vi "S4GUI.vi"(7 "Tab ObsEng":enum32{"Obs", "CCD modes", "Guider", "Eng"}(tab)) -> ()   [LabVIEW 2018] (continued)
                    n2231 = call-dynamic "save config.vi"("error in (no error)"=w4233, "file config"="lastsaved.cfg", "Channel in"=w4227) -> ("error out"=w4232:errorcluster, "Channel out"=w4226:refnum<class "Channel.lvclass">)  [unwired: 7 in]
                    n2232 = call-dynamic "Read State Machine.vi"("error in (no error)"=w4232, "Device in"=w4226) -> ("error out"=w4236:errorcluster, "State Machine.lvclass"=w4224:refnum<class "State Machine.lvclass">, "Device out"=w4225:refnum<class "Channel.lvclass">)  [unwired: 7 in]
                    n2233 = call-dynamic "Write State.vi"("error in (no error)"=w4236, "State"=60, "State Machine in"=w4224) -> ("error out"=w4235:errorcluster, "State Machine out"=w4223:refnum<class "State Machine.lvclass">)  [unwired: 7 in]
                    n2234 = call-dynamic "Write State Machine.vi"("error in (no error)"=w4235, "State Machine.lvclass"=w4223, "Device in"=w4225) -> ("error out"=w4221:errorcluster, "Device out"=w4222:refnum<class "Channel.lvclass">)  [unwired: 7 in]
                    n2235 = call-dynamic "Write Channel.vi"("error in (no error)"=w4221, "Channel.lvclass"=w4222, "Acquisition in"=w4252) -> ("error out"=w4217:errorcluster, "Acquisition out"=w4218:refnum<class "Acquisition.lvclass">)  [unwired: 7 in]
                  }
                }
                n2236 = call-dynamic "Write AcquisitionA.vi"("error in (no error)"=w4188, "Acquisition.lvclass"=w4189, "S4ACS_GUI in"=w4190) -> ("error out"=w4179:errorcluster, "S4ACS_GUI out"=w4194:refnum<class "S4GUI.lvclass">)  [unwired: 7 in]
                n2237 = call "Write AcquisitionB.vi"("error in (no error)"=w4186, "Acquisition.lvclass"=w4187, "S4ACS_GUI in"=w4194) -> ("error out"=w4178:errorcluster, "S4ACS_GUI out"=w4193:refnum<class "S4GUI.lvclass">)  [unwired: 7 in]
                n2238 = call-dynamic "Write AcquisitionC.vi"("error in (no error)"=w4184, "Acquisition.lvclass"=w4185, "S4ACS_GUI in"=w4193) -> ("error out"=w4177:errorcluster, "S4ACS_GUI out"=w4192:refnum<class "S4GUI.lvclass">)  [unwired: 7 in]
                n2239 = call-dynamic "Write AcquisitionD.vi"("error in (no error)"=w4182, "Acquisition.lvclass"=w4183, "S4ACS_GUI in"=w4192) -> ("error out"=w4176:errorcluster, "S4ACS_GUI out"=w4191:refnum<class "S4GUI.lvclass">)  [unwired: 7 in]
                n2240 = Merge Errors(w4179, w4178, w4177, w4176) -> (w4175:errorcluster)
              }
            }
            n2241 = call-dynamic "Read prev ciclos.vi"("error in (no error)"=w4162, "S4GUI in"=w4163) -> ("error out"=w4160:errorcluster, "prev ciclos"=w4159:u32, "S4GUI out"=w4161:refnum<class "S4GUI.lvclass">)  [unwired: 7 in]
            n2242 = property on="#Cycles Done" class="Slide (strict)"("Scale.Maximum"=w4159, "Scale.Minimum"=0.0 ("Scale.Range:Minimum")) -> ()  [unwired: 2 in, 2 out]
            n2243 = local write "# Cycles"(w4159) -> ()
          }
          frame 0, Default {
            # "Async mode: Os canais são configurados com Trigger Interno para Fotometria ou Trigger Externo para Polarimetria (independentemente do status do SyncBox)"
            # "Aynchronous:"
            n2244 = call-dynamic "Read AcquisitionC.vi"("error in (no error)"=w4394, "S4ACS_GUI in"=w4393) -> ("error out"=w4398:errorcluster, "Acquisition.lvclass"=w4397:refnum<class "Acquisition.lvclass">)  [unwired: 7 in, 1 out]
            n2245 = call "Read AcquisitionB.vi"("error in (no error)"=w4394, "S4ACS_GUI in"=w4393) -> ("error out"=w4399:errorcluster, "Acquisition.lvclass"=w4400:refnum<class "Acquisition.lvclass">)  [unwired: 7 in, 1 out]
            n2246 = call-dynamic "Read AcquisitionA.vi"("error in (no error)"=w4394, "S4ACS_GUI in"=w4393) -> ("error out"=w4401:errorcluster, "Acquisition.lvclass"=w4402:refnum<class "Acquisition.lvclass">, "S4ACS_GUI out"=w4383:refnum<class "S4GUI.lvclass">)  [unwired: 7 in]
            n2247 = case shown="True" w4374 {
              tunnel: [u8 0 ("SHUTTER_MODE") w4417] -> w4373
              tunnel: w4372 -> [_ w4420]
              frame False {
                # "Fotom."
                # "Internal"
              }
              frame True {
                # "exp mode?"
                # "Internal"
                # "Polar."
                # "Ext. Start"
                n2248 = Select(t=u8 0, s=w4420, f=u8 6 ("SHUTTER_MODE")) -> (s? t:f=w4417:u8)
              }
            }
            n2249 = call-dynamic "Read AcquisitionD.vi"("error in (no error)"=w4394, "S4ACS_GUI in"=w4393) -> ("error out"=w4395:errorcluster, "Acquisition.lvclass"=w4396:refnum<class "Acquisition.lvclass">)  [unwired: 7 in, 1 out]
            n2250 = call "Read connection.vi"("error in (no error)"=w4398, "Server in"=w4397) -> ("error out"=w4407:errorcluster, "connection"=w4406:bool, "Server out"=w4408:refnum<class "Acquisition.lvclass">)  [unwired: 7 in]
            n2251 = call "Read connection.vi"("error in (no error)"=w4399, "Server in"=w4400) -> ("error out"=w4410:errorcluster, "connection"=w4409:bool, "Server out"=w4411:refnum<class "Acquisition.lvclass">)  [unwired: 7 in]
            n2252 = call "Read connection.vi"("error in (no error)"=w4395, "Server in"=w4396) -> ("error out"=w4404:errorcluster, "connection"=w4403:bool, "Server out"=w4405:refnum<class "Acquisition.lvclass">)  [unwired: 7 in]
            n2253 = call "Read connection.vi"("error in (no error)"=w4401, "Server in"=w4402) -> ("error out"=w4413:errorcluster, "connection"=w4412:bool, "Server out"=w4414:refnum<class "Acquisition.lvclass">)  [unwired: 7 in]
            n2254 = case shown="True" w4406 {
              tunnel: w4408 -> [w4465 w4476]
              tunnel: w4407 -> [w4464 w4475]
              tunnel: [w4465 w4474] -> w4378
              tunnel: [w4464 w4473] -> w4377
              tunnel: w4373 -> [_ w4472]
              frame False {
              }
              frame True {
                # "nome do arquivo .cfg"
                # "seção no arquivo .cfg"
                n2255 = call-dynamic "Read Channel.vi"("error in (no error)"=w4475, "Acquisition in"=w4476) -> ("error out"=w4480:errorcluster, "Channel.lvclass"=w4479:refnum<class "Channel.lvclass">, "Acquisition out"=w4478:refnum<class "Acquisition.lvclass">)  [unwired: 7 in]
                n2256 = call-dynamic "Read Interface.vi"("error in (no error)"=w4480, "Channel in"=w4479) -> ("error out"=w4487:errorcluster, "Interface.lvclass"=w4488:refnum<class "Interface.lvclass">, "Channel out"=w4477:refnum<class "Channel.lvclass">)  [unwired: 7 in]
                n2257 = call-dynamic "Get CCD_Config.vi"("error in (no error)"=w4487, "Interface in"=w4488) -> ("error out"=w4485:errorcluster, "output cluster"=w4484:T31, "Interface out"=w4489:refnum<class "Interface.lvclass">)  [unwired: 7 in]
                n2258 = Bundle By Name(cluster=w4484, "TRIGGER_MODE"=w4472) -> (w4486:T31)
                n2259 = call-dynamic "Set CCD_Config.vi"("error in (no error)"=w4485, "input cluster"=w4486, "Interface in"=w4489) -> ("error out"=w4483:errorcluster, "Interface out"=w4490:refnum<class "Interface.lvclass">)  [unwired: 7 in]
                n2260 = Flatten To String(anything=w4486, error in (no error)=w4483) -> (data string=w4481:string, error out=w4482:errorcluster)  [unwired: 2 in, 1 out]
                n2261 = call "Write flatted cluster.vi"("error in (no error)"=w4482, "flatted cluster"=w4481, "Interface in"=w4490) -> ("error out"=w4492:errorcluster, "Interface out"=w4491:refnum<class "Interface.lvclass">)  [unwired: 7 in]
                n2262 = call-dynamic "Write Interface.vi"("error in (no error)"=w4492, "Interface.lvclass"=w4491, "Channel in"=w4477) -> ("error out"=w4498:errorcluster, "Channel out"=w4499:refnum<class "Channel.lvclass">)  [unwired: 7 in]
                n2263 = call "Write section_name.vi"("error in (no error)"=w4498, "section_name"="CCD_ACS3", "Channel in"=w4499) -> ("error out"=w4496:errorcluster, "Channel out"=w4502:refnum<class "Channel.lvclass">)  [unwired: 7 in]
                n2264 = call-dynamic "save config.vi"("error in (no error)"=w4496, "file config"="lastsaved.cfg", "Channel in"=w4502) -> ("error out"=w4497:errorcluster, "Channel out"=w4503:refnum<class "Channel.lvclass">)  [unwired: 7 in]
                n2265 = call-dynamic "Read State Machine.vi"("error in (no error)"=w4497, "Device in"=w4503) -> ("error out"=w4493:errorcluster, "State Machine.lvclass"=w4505:refnum<class "State Machine.lvclass">, "Device out"=w4504:refnum<class "Channel.lvclass">)  [unwired: 7 in]
                n2266 = call-dynamic "Write State.vi"("error in (no error)"=w4493, "State"=60, "State Machine in"=w4505) -> ("error out"=w4494:errorcluster, "State Machine out"=w4506:refnum<class "State Machine.lvclass">)  [unwired: 7 in]
                n2267 = call-dynamic "Write State Machine.vi"("error in (no error)"=w4494, "State Machine.lvclass"=w4506, "Device in"=w4504) -> ("error out"=w4470:errorcluster, "Device out"=w4471:refnum<class "Channel.lvclass">)  [unwired: 7 in]
                n2268 = call-dynamic "Read prev ciclos.vi"("error in (no error)"=w4470, "Channel in"=w4471) -> ("error out"=w4468:errorcluster, "prev ciclos"=w4466:u32, "Channel out"=w4469:refnum<class "Channel.lvclass">)  [unwired: 7 in]
                n2269 = local write "#cycles ch3"(w4466) -> ()
                n2270 = property on="Cycles Done ch3" class="Slide (strict)"("Scale.Maximum"=w4466, "Scale.Minimum"=0.0 ("Scale.Range:Minimum")) -> ()  [unwired: 2 in, 2 out]
                n2271 = call-dynamic "Write Channel.vi"("error in (no error)"=w4468, "Channel.lvclass"=w4469, "Acquisition in"=w4478) -> ("error out"=w4473:errorcluster, "Acquisition out"=w4474:refnum<class "Acquisition.lvclass">)  [unwired: 7 in]
              }
            }
            n2272 = case shown="True" w4403 {
              tunnel: w4405 -> [w4422 w4433]
              tunnel: w4404 -> [w4421 w4432]
              tunnel: [w4422 w4431] -> w4376
              tunnel: [w4421 w4430] -> w4375
              tunnel: w4373 -> [_ w4429]
              frame False {
              }
              frame True {
                # "nome do arquivo .cfg"
                # "seção no arquivo .cfg"
                n2273 = call-dynamic "Read Channel.vi"("error in (no error)"=w4432, "Acquisition in"=w4433) -> ("error out"=w4460:errorcluster, "Channel.lvclass"=w4461:refnum<class "Channel.lvclass">, "Acquisition out"=w4462:refnum<class "Acquisition.lvclass">)  [unwired: 7 in]
                n2274 = call-dynamic "Read Interface.vi"("error in (no error)"=w4460, "Channel in"=w4461) -> ("error out"=w4453:errorcluster, "Interface.lvclass"=w4452:refnum<class "Interface.lvclass">, "Channel out"=w4463:refnum<class "Channel.lvclass">)  [unwired: 7 in]
                n2275 = call-dynamic "Get CCD_Config.vi"("error in (no error)"=w4453, "Interface in"=w4452) -> ("error out"=w4455:errorcluster, "output cluster"=w4456:T31, "Interface out"=w4451:refnum<class "Interface.lvclass">)  [unwired: 7 in]
                n2276 = Bundle By Name(cluster=w4456, "TRIGGER_MODE"=w4429) -> (w4454:T31)
                n2277 = call-dynamic "Set CCD_Config.vi"("error in (no error)"=w4455, "input cluster"=w4454, "Interface in"=w4451) -> ("error out"=w4457:errorcluster, "Interface out"=w4450:refnum<class "Interface.lvclass">)  [unwired: 7 in]
                n2278 = Flatten To String(anything=w4454, error in (no error)=w4457) -> (data string=w4459:string, error out=w4458:errorcluster)  [unwired: 2 in, 1 out]
                n2279 = call "Write flatted cluster.vi"("error in (no error)"=w4458, "flatted cluster"=w4459, "Interface in"=w4450) -> ("error out"=w4448:errorcluster, "Interface out"=w4449:refnum<class "Interface.lvclass">)  [unwired: 7 in]
                n2280 = call-dynamic "Write Interface.vi"("error in (no error)"=w4448, "Interface.lvclass"=w4449, "Channel in"=w4463) -> ("error out"=w4442:errorcluster, "Channel out"=w4441:refnum<class "Channel.lvclass">)  [unwired: 7 in]
                n2281 = call "Write section_name.vi"("error in (no error)"=w4442, "section_name"="CCD_ACS4", "Channel in"=w4441) -> ("error out"=w4444:errorcluster, "Channel out"=w4438:refnum<class "Channel.lvclass">)  [unwired: 7 in]
                n2282 = call-dynamic "save config.vi"("error in (no error)"=w4444, "file config"="lastsaved.cfg", "Channel in"=w4438) -> ("error out"=w4443:errorcluster, "Channel out"=w4437:refnum<class "Channel.lvclass">)  [unwired: 7 in]
                n2283 = call-dynamic "Read State Machine.vi"("error in (no error)"=w4443, "Device in"=w4437) -> ("error out"=w4447:errorcluster, "State Machine.lvclass"=w4435:refnum<class "State Machine.lvclass">, "Device out"=w4436:refnum<class "Channel.lvclass">)  [unwired: 7 in]
                n2284 = call-dynamic "Write State.vi"("error in (no error)"=w4447, "State"=60, "State Machine in"=w4435) -> ("error out"=w4446:errorcluster, "State Machine out"=w4434:refnum<class "State Machine.lvclass">)  [unwired: 7 in]
                n2285 = call-dynamic "Write State Machine.vi"("error in (no error)"=w4446, "State Machine.lvclass"=w4434, "Device in"=w4436) -> ("error out"=w4427:errorcluster, "Device out"=w4428:refnum<class "Channel.lvclass">)  [unwired: 7 in]
                n2286 = call-dynamic "Read prev ciclos.vi"("error in (no error)"=w4427, "Channel in"=w4428) -> ("error out"=w4425:errorcluster, "prev ciclos"=w4423:u32, "Channel out"=w4426:refnum<class "Channel.lvclass">)  [unwired: 7 in]
                n2287 = local write "#cycles ch4"(w4423) -> ()
                n2288 = property on="Cycles Done ch4" class="Slide (strict)"("Scale.Maximum"=w4423, "Scale.Minimum"=0.0 ("Scale.Range:Minimum")) -> ()  [unwired: 2 in, 2 out]
                n2289 = call-dynamic "Write Channel.vi"("error in (no error)"=w4425, "Channel.lvclass"=w4426, "Acquisition in"=w4462) -> ("error out"=w4430:errorcluster, "Acquisition out"=w4431:refnum<class "Acquisition.lvclass">)  [unwired: 7 in]
              }
            }
            n2290 = case shown="True" w4409 {
              tunnel: w4411 -> [w4508 w4519]
              tunnel: w4410 -> [w4507 w4518]
              tunnel: [w4508 w4517] -> w4380
              tunnel: [w4507 w4516] -> w4379
              tunnel: w4373 -> [_ w4515]
              frame False {
              }
              frame True {
                # "nome do arquivo .cfg"
                # "seção no arquivo .cfg"
                n2291 = call-dynamic "Read Channel.vi"("error in (no error)"=w4518, "Acquisition in"=w4519) -> ("error out"=w4523:errorcluster, "Channel.lvclass"=w4522:refnum<class "Channel.lvclass">, "Acquisition out"=w4521:refnum<class "Acquisition.lvclass">)  [unwired: 7 in]
                n2292 = call-dynamic "Read Interface.vi"("error in (no error)"=w4523, "Channel in"=w4522) -> ("error out"=w4530:errorcluster, "Interface.lvclass"=w4531:refnum<class "Interface.lvclass">, "Channel out"=w4520:refnum<class "Channel.lvclass">)  [unwired: 7 in]
                n2293 = call-dynamic "Get CCD_Config.vi"("error in (no error)"=w4530, "Interface in"=w4531) -> ("error out"=w4528:errorcluster, "output cluster"=w4527:T31, "Interface out"=w4532:refnum<class "Interface.lvclass">)  [unwired: 7 in]
                n2294 = Bundle By Name(cluster=w4527, "TRIGGER_MODE"=w4515) -> (w4529:T31)
                n2295 = call-dynamic "Set CCD_Config.vi"("error in (no error)"=w4528, "input cluster"=w4529, "Interface in"=w4532) -> ("error out"=w4526:errorcluster, "Interface out"=w4533:refnum<class "Interface.lvclass">)  [unwired: 7 in]
                n2296 = Flatten To String(anything=w4529, error in (no error)=w4526) -> (data string=w4524:string, error out=w4525:errorcluster)  [unwired: 2 in, 1 out]
                n2297 = call "Write flatted cluster.vi"("error in (no error)"=w4525, "flatted cluster"=w4524, "Interface in"=w4533) -> ("error out"=w4535:errorcluster, "Interface out"=w4534:refnum<class "Interface.lvclass">)  [unwired: 7 in]
                n2298 = call-dynamic "Write Interface.vi"("error in (no error)"=w4535, "Interface.lvclass"=w4534, "Channel in"=w4520) -> ("error out"=w4541:errorcluster, "Channel out"=w4542:refnum<class "Channel.lvclass">)  [unwired: 7 in]
                n2299 = call "Write section_name.vi"("error in (no error)"=w4541, "section_name"="CCD_ACS2", "Channel in"=w4542) -> ("error out"=w4539:errorcluster, "Channel out"=w4545:refnum<class "Channel.lvclass">)  [unwired: 7 in]
                n2300 = call-dynamic "save config.vi"("error in (no error)"=w4539, "file config"="lastsaved.cfg", "Channel in"=w4545) -> ("error out"=w4540:errorcluster, "Channel out"=w4546:refnum<class "Channel.lvclass">)  [unwired: 7 in]
                n2301 = call-dynamic "Read State Machine.vi"("error in (no error)"=w4540, "Device in"=w4546) -> ("error out"=w4536:errorcluster, "State Machine.lvclass"=w4548:refnum<class "State Machine.lvclass">, "Device out"=w4547:refnum<class "Channel.lvclass">)  [unwired: 7 in]
                n2302 = call-dynamic "Write State.vi"("error in (no error)"=w4536, "State"=60, "State Machine in"=w4548) -> ("error out"=w4537:errorcluster, "State Machine out"=w4549:refnum<class "State Machine.lvclass">)  [unwired: 7 in]
                n2303 = call-dynamic "Write State Machine.vi"("error in (no error)"=w4537, "State Machine.lvclass"=w4549, "Device in"=w4547) -> ("error out"=w4513:errorcluster, "Device out"=w4514:refnum<class "Channel.lvclass">)  [unwired: 7 in]
                n2304 = call-dynamic "Read prev ciclos.vi"("error in (no error)"=w4513, "Channel in"=w4514) -> ("error out"=w4511:errorcluster, "prev ciclos"=w4509:u32, "Channel out"=w4512:refnum<class "Channel.lvclass">)  [unwired: 7 in]
                n2305 = local write "#cycles ch2"(w4509) -> ()
                n2306 = property on="Cycles Done ch2" class="Slide (strict)"("Scale.Maximum"=w4509, "Scale.Minimum"=0.0 ("Scale.Range:Minimum")) -> ()  [unwired: 2 in, 2 out]
                n2307 = call-dynamic "Write Channel.vi"("error in (no error)"=w4511, "Channel.lvclass"=w4512, "Acquisition in"=w4521) -> ("error out"=w4516:errorcluster, "Acquisition out"=w4517:refnum<class "Acquisition.lvclass">)  [unwired: 7 in]
              }
            }
            n2308 = case shown="True" w4412 {
              tunnel: [w4550 w4588] -> w4381
              tunnel: [w4551 w4587] -> w4382
              tunnel: w4414 -> [w4551 w4560]
              tunnel: w4413 -> [w4550 w4559]
              tunnel: w4373 -> [_ w4558]
              frame False {
              }
              frame True {
                # "nome do arquivo .cfg"
                # "seção no arquivo .cfg"
                n2309 = call-dynamic "Read Channel.vi"("error in (no error)"=w4559, "Acquisition in"=w4560) -> ("error out"=w4589:errorcluster, "Channel.lvclass"=w4590:refnum<class "Channel.lvclass">, "Acquisition out"=w4591:refnum<class "Acquisition.lvclass">)  [unwired: 7 in]
                n2310 = call-dynamic "Read Interface.vi"("error in (no error)"=w4589, "Channel in"=w4590) -> ("error out"=w4580:errorcluster, "Interface.lvclass"=w4579:refnum<class "Interface.lvclass">, "Channel out"=w4592:refnum<class "Channel.lvclass">)  [unwired: 7 in]
                n2311 = call-dynamic "Get CCD_Config.vi"("error in (no error)"=w4580, "Interface in"=w4579) -> ("error out"=w4582:errorcluster, "output cluster"=w4583:T31, "Interface out"=w4578:refnum<class "Interface.lvclass">)  [unwired: 7 in]
                n2312 = Bundle By Name(cluster=w4583, "TRIGGER_MODE"=w4558) -> (w4581:T31)
                n2313 = call-dynamic "Set CCD_Config.vi"("error in (no error)"=w4582, "input cluster"=w4581, "Interface in"=w4578) -> ("error out"=w4584:errorcluster, "Interface out"=w4577:refnum<class "Interface.lvclass">)  [unwired: 7 in]
                n2314 = Flatten To String(anything=w4581, error in (no error)=w4584) -> (data string=w4586:string, error out=w4585:errorcluster)  [unwired: 2 in, 1 out]
                n2315 = call "Write flatted cluster.vi"("error in (no error)"=w4585, "flatted cluster"=w4586, "Interface in"=w4577) -> ("error out"=w4575:errorcluster, "Interface out"=w4576:refnum<class "Interface.lvclass">)  [unwired: 7 in]
                n2316 = call-dynamic "Write Interface.vi"("error in (no error)"=w4575, "Interface.lvclass"=w4576, "Channel in"=w4592) -> ("error out"=w4570:errorcluster, "Channel out"=w4569:refnum<class "Channel.lvclass">)  [unwired: 7 in]
                n2317 = call "Write section_name.vi"("error in (no error)"=w4570, "section_name"="CCD_ACS1", "Channel in"=w4569) -> ("error out"=w4571:errorcluster, "Channel out"=w4566:refnum<class "Channel.lvclass">)  [unwired: 7 in]
                n2318 = call-dynamic "save config.vi"("error in (no error)"=w4571, "file config"="lastsaved.cfg", "Channel in"=w4566) -> ("error out"=w4561:errorcluster, "Channel out"=w4562:refnum<class "Channel.lvclass">)  [unwired: 7 in]
                n2319 = call-dynamic "Read State Machine.vi"("error in (no error)"=w4561, "Device in"=w4562) -> ("error out"=w4574:errorcluster, "State Machine.lvclass"=w4564:refnum<class "State Machine.lvclass">, "Device out"=w4565:refnum<class "Channel.lvclass">)  [unwired: 7 in]
                n2320 = call-dynamic "Write State.vi"("error in (no error)"=w4574, "State"=60, "State Machine in"=w4564) -> ("error out"=w4573:errorcluster, "State Machine out"=w4563:refnum<class "State Machine.lvclass">)  [unwired: 7 in]
                n2321 = call-dynamic "Write State Machine.vi"("error in (no error)"=w4573, "State Machine.lvclass"=w4563, "Device in"=w4565) -> ("error out"=w4556:errorcluster, "Device out"=w4557:refnum<class "Channel.lvclass">)  [unwired: 7 in]
                n2322 = call-dynamic "Read prev ciclos.vi"("error in (no error)"=w4556, "Channel in"=w4557) -> ("error out"=w4554:errorcluster, "prev ciclos"=w4552:u32, "Channel out"=w4555:refnum<class "Channel.lvclass">)  [unwired: 7 in]
                n2323 = local write "#cycles ch1"(w4552) -> ()
                n2324 = property on="Cycles Done ch1" class="Slide (strict)"("Scale.Maximum"=w4552, "Scale.Minimum"=0.0 ("Scale.Range:Minimum")) -> ()  [unwired: 2 in, 2 out]
                n2325 = call-dynamic "Write Channel.vi"("error in (no error)"=w4554, "Channel.lvclass"=w4555, "Acquisition in"=w4591) -> ("error out"=w4588:errorcluster, "Acquisition out"=w4587:refnum<class "Acquisition.lvclass">)  [unwired: 7 in]
              }
            }
            n2326 = call-dynamic "Write AcquisitionA.vi"("error in (no error)"=w4381, "Acquisition.lvclass"=w4382, "S4ACS_GUI in"=w4383) -> ("error out"=w4389:errorcluster, "S4ACS_GUI out"=w4392:refnum<class "S4GUI.lvclass">)  [unwired: 7 in]
            n2327 = call "Write AcquisitionB.vi"("error in (no error)"=w4379, "Acquisition.lvclass"=w4380, "S4ACS_GUI in"=w4392) -> ("error out"=w4388:errorcluster, "S4ACS_GUI out"=w4391:refnum<class "S4GUI.lvclass">)  [unwired: 7 in]
            n2328 = call-dynamic "Write AcquisitionC.vi"("error in (no error)"=w4377, "Acquisition.lvclass"=w4378, "S4ACS_GUI in"=w4391) -> ("error out"=w4387:errorcluster, "S4ACS_GUI out"=w4390:refnum<class "S4GUI.lvclass">)  [unwired: 7 in]
            n2329 = call-dynamic "Write AcquisitionD.vi"("error in (no error)"=w4375, "Acquisition.lvclass"=w4376, "S4ACS_GUI in"=w4390) -> ("error out"=w4386:errorcluster, "S4ACS_GUI out"=w4385:refnum<class "S4GUI.lvclass">)  [unwired: 7 in]
            n2330 = Merge Errors(w4389, w4388, w4387, w4386) -> (w4384:errorcluster)
          }
        }
        n2331 = Concatenate Strings(w4137, " MODE SELECTED" ("User Event")) -> (w4142:string)
        n2332 = call-dynamic "Write sync.vi"("error in (no error)"=w4155, "sync"=w4157, "S4ACS_GUI in"=w4156) -> ("error out"=w4140:errorcluster, "S4ACS_GUI out"=w4141:refnum<class "S4GUI.lvclass">)  [unwired: 7 in]
        n2333 = call-dynamic "Write User Event.vi"("error in (no error)"=w4140, "User Event"=w4142, "S4GUI in"=w4141) -> ("error out"=w4138:errorcluster, "S4GUI out"=w4139:refnum<class "S4GUI.lvclass">)  [unwired: 7 in]
      }
      event "SendExpose": Value Change {
        n2334 = event-data() -> ("NewVal"=w4593:bool)  [unwired: 1 in]
        n2335 = disable-structure shown="Enabled" {
          disable-tunnel: w4593 -> [w4731 w4732]
          disable-tunnel: [w4730 w4732] -> w4594
          frame Disabled {
            n2336 = Not(x=w4731) -> (.not. x?=w4730:bool)
          }
          frame Enabled {
          }
        }
        n2337 = disable-structure shown="Enabled" {
          disable-tunnel: w4678 -> [w4693 w4729]
          disable-tunnel: w4677 -> [w4684 w4728]
          disable-tunnel: [w4681 w4729] -> w4596
          disable-tunnel: [w4680 w4728] -> w4595
          disable-tunnel: w4593 -> [w4679 _]
          frame Disabled {
            n2338 = call-dynamic "Read Sync Box.lvclass.vi"("error in (no error)"=w4684, "SPARC4_AC in"=w4693) -> ("error out"=w4686:errorcluster, "Sync Box.lvclass"=w4692:refnum<class "Sync Box.lvclass">, "SPARC4_AC out"=w4689:refnum<class "S4GUI.lvclass">)  [unwired: 7 in]
            n2339 = call-dynamic "Read Stream.vi"("error in (no error)"=w4686, "Server in"=w4692) -> ("error out"=w4685:errorcluster, "Stream.lvclass"=w4694:refnum<class "Stream.lvclass">, "Server out"=w4683:refnum<class "Sync Box.lvclass">)  [unwired: 7 in]
            n2340 = case shown="True" w4679 {
              tunnel: [w4697 w4714] -> w4687
              tunnel: w4694 -> [w4699 w4704]
              tunnel: [w4698 w4710] -> w4691
              tunnel: w4685 -> [w4696 w4702]
              tunnel: w4683 -> [w4695 w4703]
              tunnel: [w4695 w4703] -> w4682
              frame False {
                n2341 = call-dynamic "End.vi"("error in (no error)"=w4696, "Stream in"=w4699) -> ("error out"=w4697:errorcluster, "Stream out"=w4698:refnum<class "Stream.lvclass">)  [unwired: 8 in]
              }
              frame True {
                w4707 = errorcluster {"status"=FALSE, "code"=0, "source"=""} ("error in (no error)")
                w4725 = FALSE ("Wait Until Done")
                w4720 = FALSE ("Wait Until Done")
                n2342 = call-dynamic "Read comfile name1.vi"("error in (no error)"=w4702, "Stream in"=w4704) -> ("error out"=w4716:errorcluster, "comfile name1"=w4717:string, "Stream out"=w4713:refnum<class "Stream.lvclass">)  [unwired: 7 in]
                n2343 = call <vilib>:"Application Directory.vi"() -> ("Application Directory"=w4722:path)
                n2344 = call <vilib>:"Application Directory.vi"() -> ("Application Directory"=w4726:path)
                n2345 = Build Path(base path=w4726, name or relative path=w4717) -> (appended path=w4727:path)
                n2346 = Open VI Reference(vi path=w4727, error in (no error)=w4716) -> (vi reference=w4719:refnum<vi>, error out=w4718:errorcluster)  [unwired: 4 in]
                n2347 = invoke class="VI" method="Run VI"(reference=w4719, error in=w4718, "Wait until done"=w4720, "Auto Dispose Ref"=w4720) -> (reference out=w4709:refnum<vi>, error out=→"error out 7":errorcluster)  [unwired: 1 in, 3 out]
                n2348 = call-dynamic "Write commfile ref1.vi"("error in (no error)"=w4707, "commfile ref1"=w4709, "Stream in"=w4713) -> ("error out"=w4701:errorcluster, "Stream out"=w4712:refnum<class "Stream.lvclass">)  [unwired: 7 in]
                n2349 = call-dynamic "Read comfile name2.vi"("error in (no error)"=w4701, "Stream in"=w4712) -> ("error out"=w4700:errorcluster, "comfile name2"=w4715:string, "Stream out"=w4711:refnum<class "Stream.lvclass">)  [unwired: 7 in]
                n2350 = Build Path(base path=w4722, name or relative path=w4715) -> (appended path=w4721:path)
                n2351 = Open VI Reference(vi path=w4721, error in (no error)=w4700) -> (vi reference=w4723:refnum<vi>, error out=w4724:errorcluster)  [unwired: 4 in]
                n2352 = invoke class="VI" method="Run VI"(reference=w4723, error in=w4724, "Wait until done"=w4725, "Auto Dispose Ref"=w4725) -> (reference out=w4708:refnum<vi>, error out=→"error out 8":errorcluster)  [unwired: 1 in, 3 out]
                n2353 = call-dynamic "Write commfile ref2.vi"("error in (no error)"=w4707, "commfile ref2"=w4708, "Stream in"=w4711) -> ("error out"=w4714:errorcluster, "Stream out"=w4710:refnum<class "Stream.lvclass">)  [unwired: 7 in]
              }
            }
            n2354 = call-dynamic "Write Stream.vi"("error in (no error)"=w4687, "Stream.lvclass"=w4691, "Server in"=w4682) -> ("error out"=w4688:errorcluster, "Server out"=w4690:refnum<class "Sync Box.lvclass">)  [unwired: 7 in]
            n2355 = call-dynamic "Write Sync Box.lvclass.vi"("error in (no error)"=w4688, "Sync Box.lvclass"=w4690, "SPARC4_AC in"=w4689) -> ("error out"=w4680:errorcluster, "SPARC4_AC out"=w4681:refnum<class "S4GUI.lvclass">)  [unwired: 7 in]
          }
          frame Enabled {
          }
        }
        n2356 = call-dynamic "Read AcquisitionC.vi"("error in (no error)"=w4595, "S4ACS_GUI in"=w4596) -> ("error out"=w4620:errorcluster, "Acquisition.lvclass"=w4621:refnum<class "Acquisition.lvclass">)  [unwired: 7 in, 1 out]
        n2357 = call-dynamic "Read AcquisitionA.vi"("error in (no error)"=w4595, "S4ACS_GUI in"=w4596) -> ("error out"=w4657:errorcluster, "Acquisition.lvclass"=w4656:refnum<class "Acquisition.lvclass">, "S4ACS_GUI out"=w4673:refnum<class "S4GUI.lvclass">)  [unwired: 7 in]
        n2358 = call "Read AcquisitionB.vi"("error in (no error)"=w4595, "S4ACS_GUI in"=w4596) -> ("error out"=w4637:errorcluster, "Acquisition.lvclass"=w4638:refnum<class "Acquisition.lvclass">)  [unwired: 7 in, 1 out]
        n2359 = call-dynamic "Read AcquisitionD.vi"("error in (no error)"=w4595, "S4ACS_GUI in"=w4596) -> ("error out"=w4603:errorcluster, "Acquisition.lvclass"=w4604:refnum<class "Acquisition.lvclass">)  [unwired: 7 in, 1 out]
        n2360 = call-dynamic "Read Channel.vi"("error in (no error)"=w4603, "Acquisition in"=w4604) -> ("error out"=w4606:errorcluster, "Channel.lvclass"=w4608:refnum<class "Channel.lvclass">, "Acquisition out"=w4617:refnum<class "Acquisition.lvclass">)  [unwired: 7 in]
        n2361 = call-dynamic "Read Channel.vi"("error in (no error)"=w4620, "Acquisition in"=w4621) -> ("error out"=w4623:errorcluster, "Channel.lvclass"=w4625:refnum<class "Channel.lvclass">, "Acquisition out"=w4634:refnum<class "Acquisition.lvclass">)  [unwired: 7 in]
        n2362 = call-dynamic "Read Channel.vi"("error in (no error)"=w4637, "Acquisition in"=w4638) -> ("error out"=w4640:errorcluster, "Channel.lvclass"=w4642:refnum<class "Channel.lvclass">, "Acquisition out"=w4651:refnum<class "Acquisition.lvclass">)  [unwired: 7 in]
        n2363 = call-dynamic "Read Channel.vi"("error in (no error)"=w4657, "Acquisition in"=w4656) -> ("error out"=w4653:errorcluster, "Channel.lvclass"=w4655:refnum<class "Channel.lvclass">, "Acquisition out"=w4666:refnum<class "Acquisition.lvclass">)  [unwired: 7 in]
        n2364 = call-dynamic "Write wait_expose.vi"("error in (no error)"=w4606, "wait_expose"=w4594, "Channel in"=w4608) -> ("error out"=w4605:errorcluster, "Channel out"=w4607:refnum<class "Channel.lvclass">)  [unwired: 7 in]
        n2365 = call-dynamic "Write wait_expose.vi"("error in (no error)"=w4623, "wait_expose"=w4594, "Channel in"=w4625) -> ("error out"=w4622:errorcluster, "Channel out"=w4624:refnum<class "Channel.lvclass">)  [unwired: 7 in]
        n2366 = call-dynamic "Write wait_expose.vi"("error in (no error)"=w4640, "wait_expose"=w4594, "Channel in"=w4642) -> ("error out"=w4639:errorcluster, "Channel out"=w4641:refnum<class "Channel.lvclass">)  [unwired: 7 in]
        n2367 = call-dynamic "Write wait_expose.vi"("error in (no error)"=w4653, "wait_expose"=w4594, "Channel in"=w4655) -> ("error out"=w4652:errorcluster, "Channel out"=w4654:refnum<class "Channel.lvclass">)  [unwired: 7 in]
        n2368 = call-dynamic "Read State Machine.vi"("error in (no error)"=w4605, "Device in"=w4607) -> ("error out"=w4616:errorcluster, "State Machine.lvclass"=w4612:refnum<class "State Machine.lvclass">, "Device out"=w4613:refnum<class "Channel.lvclass">)  [unwired: 7 in]
        n2369 = call-dynamic "Read State Machine.vi"("error in (no error)"=w4622, "Device in"=w4624) -> ("error out"=w4633:errorcluster, "State Machine.lvclass"=w4629:refnum<class "State Machine.lvclass">, "Device out"=w4630:refnum<class "Channel.lvclass">)  [unwired: 7 in]
        n2370 = call-dynamic "Read State Machine.vi"("error in (no error)"=w4639, "Device in"=w4641) -> ("error out"=w4650:errorcluster, "State Machine.lvclass"=w4646:refnum<class "State Machine.lvclass">, "Device out"=w4647:refnum<class "Channel.lvclass">)  [unwired: 7 in]
        n2371 = call-dynamic "Read State Machine.vi"("error in (no error)"=w4652, "Device in"=w4654) -> ("error out"=w4665:errorcluster, "State Machine.lvclass"=w4661:refnum<class "State Machine.lvclass">, "Device out"=w4662:refnum<class "Channel.lvclass">)  [unwired: 7 in]
        n2372 = call-dynamic "Write State.vi"("error in (no error)"=w4616, "State"=40, "State Machine in"=w4612) -> ("error out"=w4615:errorcluster, "State Machine out"=w4611:refnum<class "State Machine.lvclass">)  [unwired: 7 in]
        n2373 = call-dynamic "Write State.vi"("error in (no error)"=w4633, "State"=40, "State Machine in"=w4629) -> ("error out"=w4632:errorcluster, "State Machine out"=w4628:refnum<class "State Machine.lvclass">)  [unwired: 7 in]
        n2374 = call-dynamic "Write State.vi"("error in (no error)"=w4650, "State"=40, "State Machine in"=w4646) -> ("error out"=w4649:errorcluster, "State Machine out"=w4645:refnum<class "State Machine.lvclass">)  [unwired: 7 in]
        n2375 = call-dynamic "Write State.vi"("error in (no error)"=w4665, "State"=40, "State Machine in"=w4661) -> ("error out"=w4664:errorcluster, "State Machine out"=w4660:refnum<class "State Machine.lvclass">)  [unwired: 7 in]
        n2376 = call-dynamic "Write State Machine.vi"("error in (no error)"=w4615, "State Machine.lvclass"=w4611, "Device in"=w4613) -> ("error out"=w4609:errorcluster, "Device out"=w4610:refnum<class "Channel.lvclass">)  [unwired: 7 in]
        n2377 = call-dynamic "Write State Machine.vi"("error in (no error)"=w4632, "State Machine.lvclass"=w4628, "Device in"=w4630) -> ("error out"=w4626:errorcluster, "Device out"=w4627:refnum<class "Channel.lvclass">)  [unwired: 7 in]
        n2378 = call-dynamic "Write State Machine.vi"("error in (no error)"=w4649, "State Machine.lvclass"=w4645, "Device in"=w4647) -> ("error out"=w4643:errorcluster, "Device out"=w4644:refnum<class "Channel.lvclass">)  [unwired: 7 in]
        n2379 = call-dynamic "Write State Machine.vi"("error in (no error)"=w4664, "State Machine.lvclass"=w4660, "Device in"=w4662) -> ("error out"=w4658:errorcluster, "Device out"=w4659:refnum<class "Channel.lvclass">)  [unwired: 7 in]
        n2380 = call-dynamic "Write Channel.vi"("error in (no error)"=w4609, "Channel.lvclass"=w4610, "Acquisition in"=w4617) -> ("error out"=w4601:errorcluster, "Acquisition out"=w4602:refnum<class "Acquisition.lvclass">)  [unwired: 7 in]
        n2381 = call-dynamic "Write Channel.vi"("error in (no error)"=w4626, "Channel.lvclass"=w4627, "Acquisition in"=w4634) -> ("error out"=w4619:errorcluster, "Acquisition out"=w4618:refnum<class "Acquisition.lvclass">)  [unwired: 7 in]
        n2382 = call-dynamic "Write Channel.vi"("error in (no error)"=w4643, "Channel.lvclass"=w4644, "Acquisition in"=w4651) -> ("error out"=w4636:errorcluster, "Acquisition out"=w4635:refnum<class "Acquisition.lvclass">)  [unwired: 7 in]
        n2383 = call-dynamic "Write Channel.vi"("error in (no error)"=w4658, "Channel.lvclass"=w4659, "Acquisition in"=w4666) -> ("error out"=w4671:errorcluster, "Acquisition out"=w4672:refnum<class "Acquisition.lvclass">)  [unwired: 7 in]
        n2384 = call-dynamic "Write AcquisitionA.vi"("error in (no error)"=w4671, "Acquisition.lvclass"=w4672, "S4ACS_GUI in"=w4673) -> ("error out"=w4670:errorcluster, "S4ACS_GUI out"=w4676:refnum<class "S4GUI.lvclass">)  [unwired: 7 in]
        n2385 = call "Write AcquisitionB.vi"("error in (no error)"=w4636, "Acquisition.lvclass"=w4635, "S4ACS_GUI in"=w4676) -> ("error out"=w4669:errorcluster, "S4ACS_GUI out"=w4675:refnum<class "S4GUI.lvclass">)  [unwired: 7 in]
        n2386 = call-dynamic "Write AcquisitionC.vi"("error in (no error)"=w4619, "Acquisition.lvclass"=w4618, "S4ACS_GUI in"=w4675) -> ("error out"=w4668:errorcluster, "S4ACS_GUI out"=w4674:refnum<class "S4GUI.lvclass">)  [unwired: 7 in]
        n2387 = call-dynamic "Write AcquisitionD.vi"("error in (no error)"=w4601, "Acquisition.lvclass"=w4602, "S4ACS_GUI in"=w4674) -> ("error out"=w4667:errorcluster, "S4ACS_GUI out"=w4600:refnum<class "S4GUI.lvclass">)  [unwired: 7 in]
        n2388 = Merge Errors(w4670, w4669, w4668, w4667) -> (w4599:errorcluster)
        n2389 = call-dynamic "Write mode EXPOSE.vi"("error in (no error)"=w4599, "mode EXPOSE"=w4594, "S4GUI in"=w4600) -> ("error out"=w4597:errorcluster, "S4GUI out"=w4598:refnum<class "S4GUI.lvclass">)  [unwired: 7 in]
      }
      event "CH1on": Value Change {
        n2390 = event-data() -> ("NewVal"=w4742:bool)  [unwired: 1 in]
        n2391 = call-dynamic "Read AcquisitionA.vi"("error in (no error)"=w4756, "S4ACS_GUI in"=w4757) -> ("error out"=w4748:errorcluster, "Acquisition.lvclass"=w4753:refnum<class "Acquisition.lvclass">, "S4ACS_GUI out"=w4749:refnum<class "S4GUI.lvclass">)  [unwired: 7 in]
        n2392 = call-dynamic "Read Channel.vi"("error in (no error)"=w4748, "Acquisition in"=w4753) -> ("error out"=w4747:errorcluster, "Channel.lvclass"=w4738:refnum<class "Channel.lvclass">, "Acquisition out"=w4752:refnum<class "Acquisition.lvclass">)  [unwired: 7 in]
        n2393 = call-dynamic "Read Stream.vi"("error in (no error)"=w4747, "Server in"=w4752) -> ("error out"=w4740:errorcluster, "Stream.lvclass"=w4741:refnum<class "Stream.lvclass">, "Server out"=w4739:refnum<class "Acquisition.lvclass">)  [unwired: 7 in]
        n2394 = case shown="False" w4742 {
          selector: w4742 -> [w4758 w4780]
          tunnel: [w4764 w4784] -> w4736
          tunnel: w4741 -> [w4773 _]
          tunnel: [w4772 w4787] -> w4735
          tunnel: w4740 -> [w4759 w4781]
          tunnel: w4739 -> [w4760 w4782]
          tunnel: [w4760 w4786] -> w4734
          tunnel: w4738 -> [w4771 w4783]
          tunnel: [w4769 w4783] -> w4733
          tunnel: [w4758 w4780] -> w4737
          frame False {
            # "força FALSE nos parametros do CCD"
            n2395 = call-dynamic "Read Interface.vi"("error in (no error)"=w4759, "Channel in"=w4771) -> ("error out"=w4768:errorcluster, "Interface.lvclass"=w4762:refnum<class "Interface.lvclass">, "Channel out"=w4770:refnum<class "Channel.lvclass">)  [unwired: 7 in]
            n2396 = disable-structure shown="Enabled" {
              disable-tunnel: w4773 -> [w4777 w4779]
              disable-tunnel: [w4776 w4779] -> w4772
              disable-tunnel: [w4775 w4778] -> w4765
              disable-tunnel: w4759 -> [w4774 w4778]
              frame Disabled {
                n2397 = call-dynamic "End.vi"("error in (no error)"=w4774, "Stream in"=w4777) -> ("error out"=w4775:errorcluster, "Stream out"=w4776:refnum<class "Stream.lvclass">)  [unwired: 8 in]
              }
              frame Enabled {
              }
            }
            n2398 = call "Write Checked Params.vi"("error in (no error)"=w4768, "Checked Params"=T14 {"ACQUISITION_MODE"=FALSE, "TRIGGER_MODE"=FALSE, "READ_MODE"=FALSE, "PREAMP"=FALSE, "READOUT_RATE"=FALSE, "VERTICAL_SHIFT_SPEED"=FALSE, "EM_MODE"=FALSE, "EM_GAIN"=FALSE, "SHUTTER_MODE"=FALSE, "SHUTTER_TTL"=FALSE, "SHUTTER_OPENING_TIME"=FALSE, "SHUTTER_CLOSING_TIME"=FALSE, "VBIN"=FALSE, "HBIN"=FALSE, "INITIAL_LINE"=FALSE, "INITIAL_COLUMN"=FALSE, "FINAL_LINE"=FALSE, "FINAL_COLUMN"=FALSE, "FRAME_TRANSFER"=FALSE, "VERTICAL_CLOCK_VOLTAGE"=FALSE, "AD_CHANNEL"=FALSE}, "Interface in"=w4762) -> ("error out"=w4767:errorcluster, "Interface out"=w4761:refnum<class "Interface.lvclass">)  [unwired: 7 in]
            n2399 = call-dynamic "Write Interface.vi"("error in (no error)"=w4767, "Interface.lvclass"=w4761, "Channel in"=w4770) -> ("error out"=w4766:errorcluster, "Channel out"=w4769:refnum<class "Channel.lvclass">)  [unwired: 7 in]
            n2400 = Merge Errors(w4766, w4765) -> (w4764:errorcluster)
          }
          frame True {
            n2401 = call-dynamic "Read Stream.vi"("error in (no error)"=w4781, "Server in"=w4782) -> ("error out"=w4785:errorcluster, "Stream.lvclass"=w4788:refnum<class "Stream.lvclass">, "Server out"=w4786:refnum<class "Acquisition.lvclass">)  [unwired: 7 in]
            n2402 = disable-structure shown="Enabled" {
              disable-tunnel: w4788 -> [w4794 w4804]
              disable-tunnel: [w4793 w4804] -> w4787
              disable-tunnel: w4785 -> [w4791 w4803]
              disable-tunnel: [w4789 w4803] -> w4784
              frame Disabled {
                w4802 = FALSE ("Wait Until Done")
                n2403 = call-dynamic "Read comfile name1.vi"("error in (no error)"=w4791, "Stream in"=w4794) -> ("error out"=w4790:errorcluster, "comfile name1"=w4797:string, "Stream out"=w4792:refnum<class "Stream.lvclass">)  [unwired: 7 in]
                n2404 = call <vilib>:"Application Directory.vi"() -> ("Application Directory"=w4799:path)
                n2405 = Build Path(base path=w4799, name or relative path=w4797) -> (appended path=w4798:path)
                n2406 = Open VI Reference(vi path=w4798, error in (no error)=w4790) -> (vi reference=w4800:refnum<vi>, error out=w4801:errorcluster)  [unwired: 4 in]
                n2407 = invoke class="VI" method="Run VI"(reference=w4800, error in=w4801, "Wait until done"=w4802, "Auto Dispose Ref"=w4802) -> (reference out=w4796:refnum<vi>, error out=w4795:errorcluster)  [unwired: 1 in, 3 out]
                n2408 = call-dynamic "Write commfile ref1.vi"("error in (no error)"=w4795, "commfile ref1"=w4796, "Stream in"=w4792) -> ("error out"=w4789:errorcluster, "Stream out"=w4793:refnum<class "Stream.lvclass">)  [unwired: 7 in]
              }
              frame Enabled {
              }
            }
          }
        }
        n2409 = call-dynamic "Write Stream.vi"("error in (no error)"=w4736, "Stream.lvclass"=w4735, "Server in"=w4734) -> ("error out"=w4746:errorcluster, "Server out"=w4744:refnum<class "Acquisition.lvclass">)  [unwired: 7 in]
        n2410 = call-dynamic "Write enabled.vi"("error in (no error)"=w4746, "enabled"=w4737, "Server in"=w4744) -> ("error out"=w4745:errorcluster, "Server out"=w4743:refnum<class "Acquisition.lvclass">)  [unwired: 7 in]
        n2411 = call-dynamic "Write Channel.vi"("error in (no error)"=w4745, "Channel.lvclass"=w4733, "Acquisition in"=w4743) -> ("error out"=w4751:errorcluster, "Acquisition out"=w4750:refnum<class "Acquisition.lvclass">)  [unwired: 7 in]
        n2412 = call-dynamic "Write AcquisitionA.vi"("error in (no error)"=w4751, "Acquisition.lvclass"=w4750, "S4ACS_GUI in"=w4749) -> ("error out"=w4754:errorcluster, "S4ACS_GUI out"=w4755:refnum<class "S4GUI.lvclass">)  [unwired: 7 in]
      }
      event "CH2on": Value Change {
        n2413 = event-data() -> ("NewVal"=w4806:bool)  [unwired: 1 in]
        n2414 = call "Read AcquisitionB.vi"("error in (no error)"=w4828, "S4ACS_GUI in"=w4829) -> ("error out"=w4820:errorcluster, "Acquisition.lvclass"=w4825:refnum<class "Acquisition.lvclass">, "S4ACS_GUI out"=w4821:refnum<class "S4GUI.lvclass">)  [unwired: 7 in]
        n2415 = call-dynamic "Read Channel.vi"("error in (no error)"=w4820, "Acquisition in"=w4825) -> ("error out"=w4819:errorcluster, "Channel.lvclass"=w4814:refnum<class "Channel.lvclass">, "Acquisition out"=w4824:refnum<class "Acquisition.lvclass">)  [unwired: 7 in]
        n2416 = call-dynamic "Read Stream.vi"("error in (no error)"=w4819, "Server in"=w4824) -> ("error out"=w4810:errorcluster, "Stream.lvclass"=w4807:refnum<class "Stream.lvclass">, "Server out"=w4812:refnum<class "Acquisition.lvclass">)  [unwired: 7 in]
        n2417 = case shown="False" w4806 {
          selector: w4806 -> [w4830 w4852]
          tunnel: [w4836 w4856] -> w4809
          tunnel: w4807 -> [w4845 _]
          tunnel: [w4844 w4859] -> w4808
          tunnel: w4810 -> [w4831 w4853]
          tunnel: w4812 -> [w4832 w4854]
          tunnel: [w4832 w4858] -> w4811
          tunnel: w4814 -> [w4843 w4855]
          tunnel: [w4841 w4855] -> w4813
          tunnel: [w4830 w4852] -> w4805
          frame False {
            # "força FALSE nos parametros do CCD"
            n2418 = call-dynamic "Read Interface.vi"("error in (no error)"=w4831, "Channel in"=w4843) -> ("error out"=w4840:errorcluster, "Interface.lvclass"=w4834:refnum<class "Interface.lvclass">, "Channel out"=w4842:refnum<class "Channel.lvclass">)  [unwired: 7 in]
            n2419 = disable-structure shown="Enabled" {
              disable-tunnel: w4845 -> [w4849 w4851]
              disable-tunnel: [w4848 w4851] -> w4844
              disable-tunnel: [w4847 w4850] -> w4837
              disable-tunnel: w4831 -> [w4846 w4850]
              frame Disabled {
                n2420 = call-dynamic "End.vi"("error in (no error)"=w4846, "Stream in"=w4849) -> ("error out"=w4847:errorcluster, "Stream out"=w4848:refnum<class "Stream.lvclass">)  [unwired: 8 in]
              }
              frame Enabled {
              }
            }
            n2421 = call "Write Checked Params.vi"("error in (no error)"=w4840, "Checked Params"=T14 {"ACQUISITION_MODE"=FALSE, "TRIGGER_MODE"=FALSE, "READ_MODE"=FALSE, "PREAMP"=FALSE, "READOUT_RATE"=FALSE, "VERTICAL_SHIFT_SPEED"=FALSE, "EM_MODE"=FALSE, "EM_GAIN"=FALSE, "SHUTTER_MODE"=FALSE, "SHUTTER_TTL"=FALSE, "SHUTTER_OPENING_TIME"=FALSE, "SHUTTER_CLOSING_TIME"=FALSE, "VBIN"=FALSE, "HBIN"=FALSE, "INITIAL_LINE"=FALSE, "INITIAL_COLUMN"=FALSE, "FINAL_LINE"=FALSE, "FINAL_COLUMN"=FALSE, "FRAME_TRANSFER"=FALSE, "VERTICAL_CLOCK_VOLTAGE"=FALSE, "AD_CHANNEL"=FALSE}, "Interface in"=w4834) -> ("error out"=w4839:errorcluster, "Interface out"=w4833:refnum<class "Interface.lvclass">)  [unwired: 7 in]
            n2422 = call-dynamic "Write Interface.vi"("error in (no error)"=w4839, "Interface.lvclass"=w4833, "Channel in"=w4842) -> ("error out"=w4838:errorcluster, "Channel out"=w4841:refnum<class "Channel.lvclass">)  [unwired: 7 in]
            n2423 = Merge Errors(w4838, w4837) -> (w4836:errorcluster)
          }
          frame True {
            n2424 = call-dynamic "Read Stream.vi"("error in (no error)"=w4853, "Server in"=w4854) -> ("error out"=w4857:errorcluster, "Stream.lvclass"=w4860:refnum<class "Stream.lvclass">, "Server out"=w4858:refnum<class "Acquisition.lvclass">)  [unwired: 7 in]
            n2425 = disable-structure shown="Enabled" {
              disable-tunnel: w4860 -> [w4866 w4876]
              disable-tunnel: [w4865 w4876] -> w4859
              disable-tunnel: w4857 -> [w4863 w4875]
              disable-tunnel: [w4861 w4875] -> w4856
              frame Disabled {
                w4874 = FALSE ("Wait Until Done")
                n2426 = call-dynamic "Read comfile name1.vi"("error in (no error)"=w4863, "Stream in"=w4866) -> ("error out"=w4862:errorcluster, "comfile name1"=w4869:string, "Stream out"=w4864:refnum<class "Stream.lvclass">)  [unwired: 7 in]
                n2427 = call <vilib>:"Application Directory.vi"() -> ("Application Directory"=w4871:path)
                n2428 = Build Path(base path=w4871, name or relative path=w4869) -> (appended path=w4870:path)
                n2429 = Open VI Reference(vi path=w4870, error in (no error)=w4862) -> (vi reference=w4872:refnum<vi>, error out=w4873:errorcluster)  [unwired: 4 in]
                n2430 = invoke class="VI" method="Run VI"(reference=w4872, error in=w4873, "Wait until done"=w4874, "Auto Dispose Ref"=w4874) -> (reference out=w4868:refnum<vi>, error out=w4867:errorcluster)  [unwired: 1 in, 3 out]
                n2431 = call-dynamic "Write commfile ref1.vi"("error in (no error)"=w4867, "commfile ref1"=w4868, "Stream in"=w4864) -> ("error out"=w4861:errorcluster, "Stream out"=w4865:refnum<class "Stream.lvclass">)  [unwired: 7 in]
              }
              frame Enabled {
              }
            }
          }
        }
        n2432 = call-dynamic "Write Stream.vi"("error in (no error)"=w4809, "Stream.lvclass"=w4808, "Server in"=w4811) -> ("error out"=w4816:errorcluster, "Server out"=w4818:refnum<class "Acquisition.lvclass">)  [unwired: 7 in]
        n2433 = call-dynamic "Write enabled.vi"("error in (no error)"=w4816, "enabled"=w4805, "Server in"=w4818) -> ("error out"=w4815:errorcluster, "Server out"=w4817:refnum<class "Acquisition.lvclass">)  [unwired: 7 in]
        n2434 = call-dynamic "Write Channel.vi"("error in (no error)"=w4815, "Channel.lvclass"=w4813, "Acquisition in"=w4817) -> ("error out"=w4823:errorcluster, "Acquisition out"=w4822:refnum<class "Acquisition.lvclass">)  [unwired: 7 in]
        n2435 = call "Write AcquisitionB.vi"("error in (no error)"=w4823, "Acquisition.lvclass"=w4822, "S4ACS_GUI in"=w4821) -> ("error out"=w4826:errorcluster, "S4ACS_GUI out"=w4827:refnum<class "S4GUI.lvclass">)  [unwired: 7 in]
      }
      event "CH3 on": Value Change {
        n2436 = event-data() -> ("NewVal"=w4893:bool)  [unwired: 1 in]
        n2437 = call-dynamic "Read AcquisitionC.vi"("error in (no error)"=w4896, "S4ACS_GUI in"=w4900) -> ("error out"=w4885:errorcluster, "Acquisition.lvclass"=w4890:refnum<class "Acquisition.lvclass">, "S4ACS_GUI out"=w4886:refnum<class "S4GUI.lvclass">)  [unwired: 7 in]
        n2438 = call-dynamic "Read Channel.vi"("error in (no error)"=w4885, "Acquisition in"=w4890) -> ("error out"=w4884:errorcluster, "Channel.lvclass"=w4883:refnum<class "Channel.lvclass">, "Acquisition out"=w4889:refnum<class "Acquisition.lvclass">)  [unwired: 7 in]
        n2439 = call-dynamic "Read Stream.vi"("error in (no error)"=w4884, "Server in"=w4889) -> ("error out"=w4897:errorcluster, "Stream.lvclass"=w4901:refnum<class "Stream.lvclass">, "Server out"=w4895:refnum<class "Acquisition.lvclass">)  [unwired: 7 in]
        n2440 = case shown="False" w4893 {
          selector: w4893 -> [w4902 w4924]
          tunnel: [w4908 w4928] -> w4898
          tunnel: w4901 -> [w4917 _]
          tunnel: [w4916 w4931] -> w4899
          tunnel: w4897 -> [w4903 w4925]
          tunnel: w4895 -> [w4904 w4926]
          tunnel: [w4904 w4930] -> w4894
          tunnel: w4883 -> [w4915 w4927]
          tunnel: [w4913 w4927] -> w4882
          tunnel: [w4902 w4924] -> w4877
          frame False {
            # "força FALSE nos parametros do CCD"
            n2441 = call-dynamic "Read Interface.vi"("error in (no error)"=w4903, "Channel in"=w4915) -> ("error out"=w4912:errorcluster, "Interface.lvclass"=w4906:refnum<class "Interface.lvclass">, "Channel out"=w4914:refnum<class "Channel.lvclass">)  [unwired: 7 in]
            n2442 = disable-structure shown="Disabled" {
              disable-tunnel: w4917 -> [w4921 w4923]
              disable-tunnel: [w4920 w4923] -> w4916
              disable-tunnel: [w4919 w4922] -> w4909
              disable-tunnel: w4903 -> [w4918 w4922]
              frame Disabled {
                n2443 = call-dynamic "End.vi"("error in (no error)"=w4918, "Stream in"=w4921) -> ("error out"=w4919:errorcluster, "Stream out"=w4920:refnum<class "Stream.lvclass">)  [unwired: 8 in]
              }
              frame Enabled {
              }
            }
            n2444 = call "Write Checked Params.vi"("error in (no error)"=w4912, "Checked Params"=T14 {"ACQUISITION_MODE"=FALSE, "TRIGGER_MODE"=FALSE, "READ_MODE"=FALSE, "PREAMP"=FALSE, "READOUT_RATE"=FALSE, "VERTICAL_SHIFT_SPEED"=FALSE, "EM_MODE"=FALSE, "EM_GAIN"=FALSE, "SHUTTER_MODE"=FALSE, "SHUTTER_TTL"=FALSE, "SHUTTER_OPENING_TIME"=FALSE, "SHUTTER_CLOSING_TIME"=FALSE, "VBIN"=FALSE, "HBIN"=FALSE, "INITIAL_LINE"=FALSE, "INITIAL_COLUMN"=FALSE, "FINAL_LINE"=FALSE, "FINAL_COLUMN"=FALSE, "FRAME_TRANSFER"=FALSE, "VERTICAL_CLOCK_VOLTAGE"=FALSE, "AD_CHANNEL"=FALSE}, "Interface in"=w4906) -> ("error out"=w4911:errorcluster, "Interface out"=w4905:refnum<class "Interface.lvclass">)  [unwired: 7 in]
            n2445 = call-dynamic "Write Interface.vi"("error in (no error)"=w4911, "Interface.lvclass"=w4905, "Channel in"=w4914) -> ("error out"=w4910:errorcluster, "Channel out"=w4913:refnum<class "Channel.lvclass">)  [unwired: 7 in]
            n2446 = Merge Errors(w4910, w4909) -> (w4908:errorcluster)
          }
          frame True {
